vi "ControlP.vi"(0 "Kp":dbl=0.02, 1 "Referencia superior":dbl, 2 "Posición anterior":dbl, 3 "Coordenada X o Y":dbl, 4 "Parar":bool, 5 "Referencia":dbl, 6 "Referencia inferior":dbl) -> (7 "Posición":dbl)   [LabVIEW 2014]
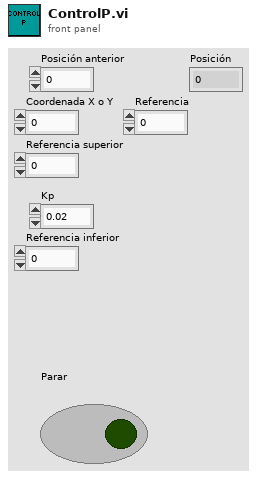
[diagram p1: front panel]
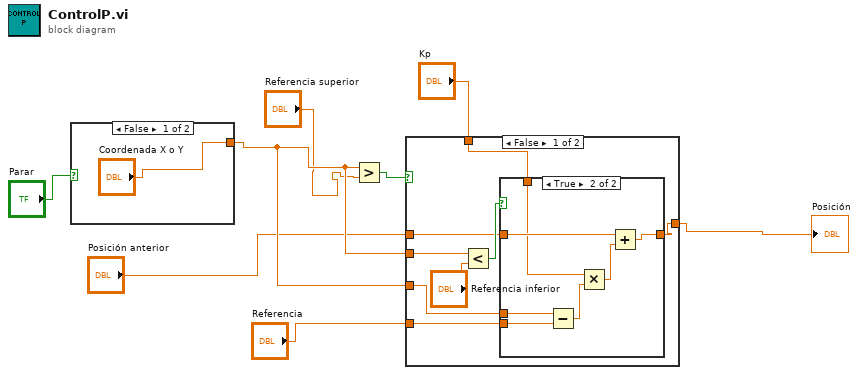
[diagram p0: block diagram]
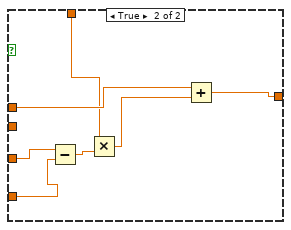
[diagram p3: hidden frame]
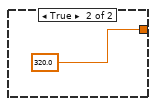
[diagram p4: hidden frame]
diagram:
  n1 = case shown="False" "Parar" {
    tunnel: ["Coordenada X o Y" 320.0] -> w8
    frame False {
    }
    frame True {
    }
  }
  n2 = Greater?(x=w8, y="Referencia superior") -> (0:w4:bool)
  n3 = case shown="False" w4 {
    tunnel: [w18 w32] -> w6
    tunnel: "Posición anterior" -> [w15 w33]
    tunnel: w8 -> [w16 _]
    tunnel: w8 -> [w14 w29]
    tunnel: "Kp" -> [w13 w28]
    tunnel: "Referencia" -> [w12 w27]
    frame False {
      n4 = Less?(x=w16, y="Referencia inferior") -> (x < y?=w17:bool)
      n5 = case shown="True" w17 {
        tunnel: [w19 w26] -> w18
        tunnel: w15 -> [w19 w24]
        tunnel: w14 -> [_ w25]
        tunnel: w13 -> [_ w21]
        tunnel: w12 -> [_ w20]
        frame False {
        }
        frame True {
          n6 = Subtract(x=w25, y=w20) -> (x-y=w23:dbl)
          n7 = Multiply(x=w21, y=w23) -> (x*y=w22:dbl)
          n8 = Add(x=w24, y=w22) -> (x+y=w26:dbl)
        }
      }
    }
    frame True {
      n9 = Subtract(x=w29, y=w27) -> (x-y=w31:dbl)
      n10 = Multiply(x=w28, y=w31) -> (x*y=w30:dbl)
      n11 = Add(x=w33, y=w30) -> (x+y=w32:dbl)
    }
  }
  "Posición" <- w6
